vi "Stop Utilization HTTP.vi"(8 "error in (no error)":errorcluster, 10 "configuration":refnum<class "NI Skyline Configuration HTTP.lvclass">, 11 "utilizationIdentifier":string) -> (0 "error out":errorcluster)   [LabVIEW 2024, in "Logger.lvclass"]
uses:
  Logger.lvclass
  <vilib>/Skyline/Configuration/Configuration HTTP_class/NI Skyline Configuration HTTP.lvclass
  <vilib>/Skyline/Configuration/Configuration HTTP_class/NI Skyline Configuration HTTP.lvclass/NI Skyline Configuration HTTP.ctl
  <vilib>/Skyline/Configuration/Configuration HTTP_class/Read Server URL.vi
  <vilib>/httpClient/PUTBuffer.vi
  <vilib>/httpClient/LabVIEWHTTPClient.lvlib
panel:
  out "URL":string
  out "JSON string":string
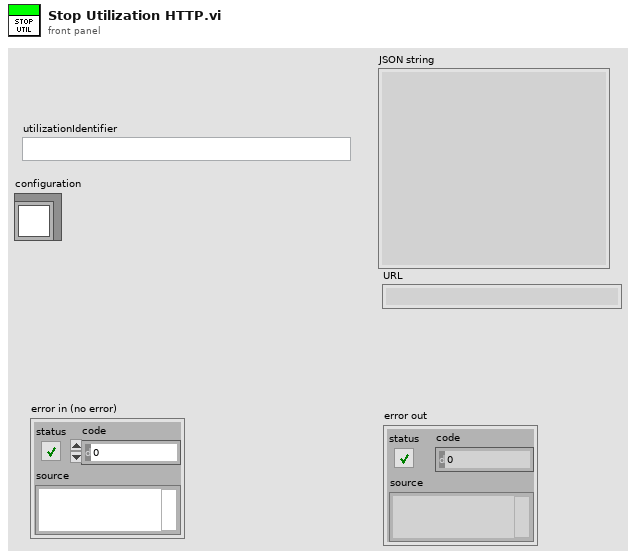
[diagram p1: front panel]
types:
  T1 = cluster{"utilizationIdentifiers":string[], "utilizationTimestamp":string}
  T2 = typedef "LabVIEWHTTPClient.lvlib/ClientHandle.ctl" = refnum<k1>
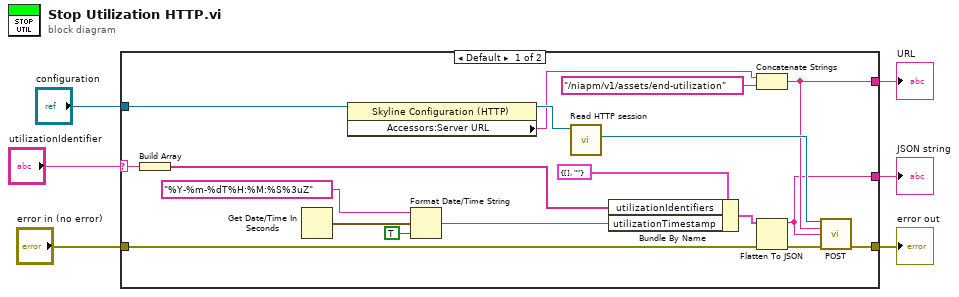
[diagram p0: block diagram]
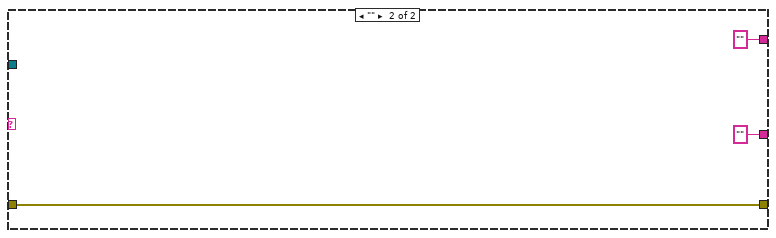
[diagram p2: hidden frame]
diagram:
  n1 = case shown="Default" "utilizationIdentifier" {
    selector: "utilizationIdentifier" -> [w7 _]
    tunnel: "error in (no error)" -> [w19 w26]
    tunnel: "configuration" -> [w18 _]
    tunnel: [w13 ""] -> w4
    tunnel: [w12 "" ("JSON string")] -> w3
    tunnel: [w10 w26] -> w2
    frame Default {
      n2 = Build Array(w7) -> (w8:string[])
      n3 = Get Date/Time In Seconds() -> (seconds since 1Jan1904=w21:timestamp)
      n4 = property class="Skyline Configuration (HTTP)"(reference=w18) -> (reference out=w17:refnum<class "NI Skyline Configuration HTTP.lvclass">, "Accessors:Server URL"=w15:string)  [unwired: 1 in, 1 out]
      n5 = Format Date/Time String(time format string (%c)="%Y-%m-%dT%H:%M:%S%3uZ", seconds (now)=w21, UTC format=TRUE) -> (date/time string=w24:string)
      n6 = call <vilib>:"Read HTTP session.vi"("HTTP configuration in"=w17) -> ("http session"=w16:T2)  [unwired: 8 in, 2 out]
      n7 = Bundle By Name(cluster=T1 {"utilizationIdentifiers"=[], "utilizationTimestamp"=""}, "utilizationIdentifiers"=w8, "utilizationTimestamp"=w24) -> (w20:T1)
      n8 = Concatenate Strings(w15, "/niapm/v1/assets/end-utilization") -> (w13:string)
      n9 = Flatten To JSON(anything=w20, error in (no error)=w19) -> (JSON string=w12:string, 11:w11:errorcluster)  [unwired: 1 in]
      n10 = call-poly <vilib>:"POST.vi"("client handle"=w16, "url"=w13, "buffer"=w12, "error in (no error)"=w11) -> ("error out"=w10:errorcluster)  [unwired: 8 in, 3 out]
    }
    frame "" {
    }
  }
  "JSON string" <- w3
  "error out" <- w2
  "URL" <- w4
